vi "GetSubVIsPath.vi"(5 "SubVIs relative path":path=path "subVIs", 6 "error in":errorcluster, 9 "RasPi Compiler in":refnum<class "RasPi Compiler.lvclass">) -> (0 "error out":errorcluster, 3 "RasPi Compiler out":refnum<class "RasPi Compiler.lvclass">, 4 "SubVIs path":path)   [LabVIEW 2014, in "Raspberry Pi Compatible Compiler for LabVIEW.lvlib" / "RasPi Compiler.lvclass"]
uses:
  RasPi Compiler.lvclass
  RasPi Compiler.lvclass/RasPi Compiler.ctl
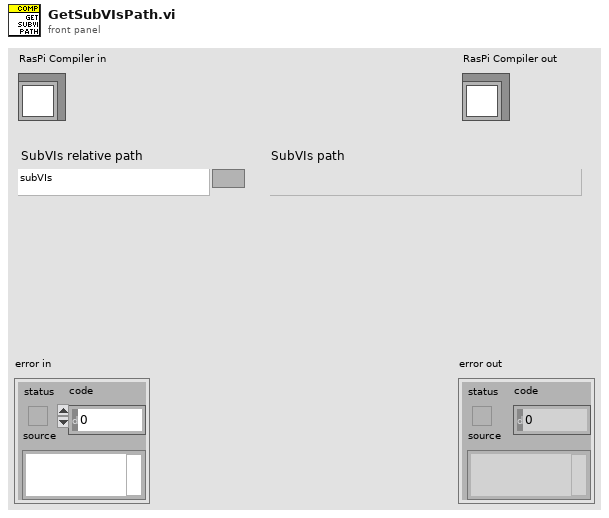
[diagram p1: front panel]
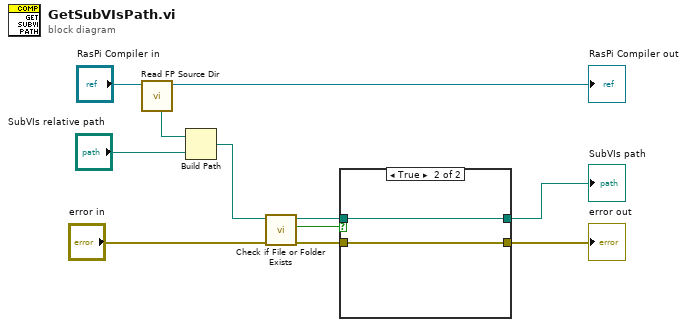
[diagram p0: block diagram]
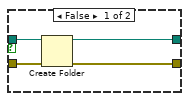
[diagram p2: hidden frame]
diagram:
  n1 = call "Read FP Source Dir.vi"("RasPi Compiler in"="RasPi Compiler in") -> ("RasPi Compiler out"=→"RasPi Compiler out":refnum<class "RasPi Compiler.lvclass">, "FP Source Dir"=w1:path)  [unwired: 7 in]
  n2 = Build Path(base path=w1, name or relative path="SubVIs relative path") -> (appended path=w10:path)
  n3 = call <vilib>:"Check if File or Folder Exists.vi"("error in (no error)"="error in", "path"=w10) -> ("error out"=w6:errorcluster, "file or folder exists?"=w8:bool, "dup path"=w7:path)  [unwired: 7 in]
  n4 = case shown="True" w8 {
    tunnel: w7 -> [w15 w17]
    tunnel: w6 -> [w14 w16]
    tunnel: [w13 w17] -> w4
    tunnel: [w12 w16] -> w5
    frame False {
      n5 = Create Folder(path (use dialog)=w15, error in=w14) -> (created path=w13:path, error out=w12:errorcluster)  [unwired: 1 in, 1 out]
    }
    frame True {
    }
  }
  "error out" <- w5
  "SubVIs path" <- w4
